vi "XY Graph Ellipse Plot.vi"(6 "angle":dbl format="%#_4g", 7 "N":i32=100, 8 "ay":dbl format="%#_4g", 9 "ax":dbl format="%#_4g", 10 "yc":dbl format="%#_4g", 11 "xc":dbl format="%#_4g") -> (3 "Ellipse":cluster{"x":dbl[], "y":dbl[]})   [LabVIEW 2021, in "XY Graph Add-Ons.lvlib"]
uses:
  XY Graph Add-Ons.lvlib
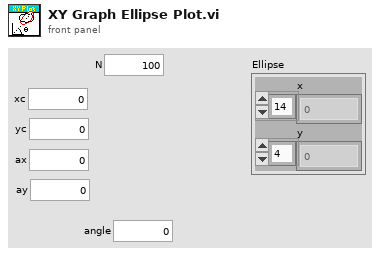
[diagram p1: front panel]
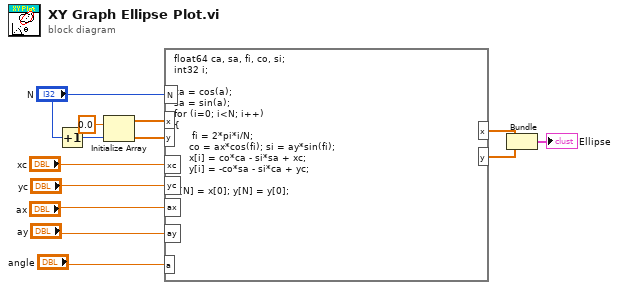
[diagram p0: block diagram]
diagram:
  n1 = Increment(x="N") -> (x+1=w11:i32)
  n2 = Initialize Array(0.0 ("element"), w11) -> (w9:dbl[])
  n3 = formula code="float64 ca, sa, fi, co, si;\nint32 i;\n\nca = cos(a);\nsa = sin(a);\nfor (i=0; i<N; i++)\n{\n      fi = 2*pi*i/N;\n     co = ax*cos(fi); si = ay*sin(fi);\n     x[i] = co*ca - si*sa + xc;\n     y[i] = -co*sa - si*ca + yc;\n}\nx[N] = x[0]; y[N] = y[0];"("a"="angle", "N"="N", "x"=w9, "y"=w9, "xc"="xc", "yc"="yc", "ax"="ax", "ay"="ay") -> ("x"=w3:dbl[], "y"=w2:dbl[])
  n4 = Bundle("x"=w3, "y"=w2) -> (→"Ellipse":cluster{"x":dbl[], "y":dbl[]})  [unwired: 1 in]
